vi "addsumedit.vi"() -> ()   [LabVIEW 2017]
panel:
  out "x+y":dbl
  out "x-y":dbl
  in  "y":dbl
  in  "x":dbl
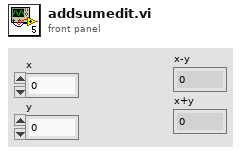
[diagram p1: front panel]
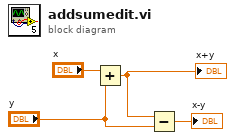
[diagram p0: block diagram]
diagram:
  n1 = Add(x="x", y="y") -> (x+y=w4:dbl)
  "x+y" <- w4
  n2 = Subtract(x=w4, y="y") -> (x-y=→"x-y":dbl)
